vi "Yscaling_raw.vi"(6 "Scaling?":bool, 10 "Y":dbl, 11 "Plane Height (m)":dbl) -> (3 "y scaled (m)":dbl, 4 "Zpos Graph (nm)":cluster{dbl, "function return":dbl})   [LabVIEW 2019]
uses:
  GlobalClicksHeight_raw.vi
  2017 FINAL/Users/brarlab/Documents/GitHub/LabView-VIs/nanonis vers/Program Files/National Instruments/LabVIEW 2019/user.lib/HapticSTM/HapticSTM.lvlib
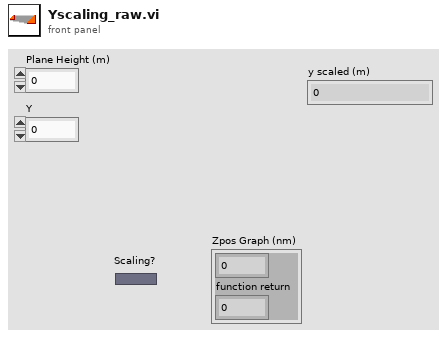
[diagram p1: front panel]
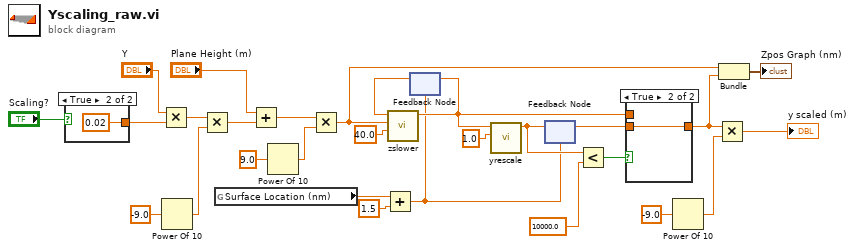
[diagram p0: block diagram]
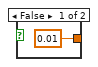
[diagram p2: hidden frame]
diagram:
  n1 = case shown="True" "Scaling?" {
    tunnel: [0.01 ("y") 0.02 ("y")] -> w1
    frame False {
    }
    frame True {
    }
  }
  n2 = Multiply(x="Y", y=w1) -> (x*y=w24:dbl)
  n3 = Power Of 10(x=-9.0) -> (10^x=w23:dbl)
  n4 = Multiply(x=w24, y=w23) -> (x*y=w25:dbl)
  n5 = global read "GlobalClicksHeight_raw.vi" "Surface Location (nm)"() -> (w6:dbl)
  n6 = Add(x="Plane Height (m)", y=w25) -> (x+y=w28:dbl)
  n7 = Power Of 10(x=9.0) -> (10^x=w27:dbl)
  n8 = Multiply(x=w28, y=w27) -> (x*y=w9:dbl)
  n9 = Add(x=w6, y=1.5) -> (x+y=w4:dbl)
  n10 = feedback #1(w4) -> (w11:dbl)
  n11 = call "zslower.vi"("maxvel"=40.0, "labview_zpos_write"=w9, "nanonis_zpos_read"=w11) -> ("function return"=w7:dbl)  [unwired: 8 in]
  n12 = feedback-in #1(w7) -> ()
  n13 = call "yrescale.vi"("scalingfactor"=1.0, "ylabview"=w7) -> ("function return"=w8:dbl)  [unwired: 9 in]
  n14 = feedback-in #2(w8) -> ()
  n15 = feedback #2(w4) -> (w13:dbl)
  n16 = Less?(x=w8, y=10000.0) -> (x < y?=w14:bool)
  n17 = case shown="True" w14 {
    tunnel: [w31 w32] -> w3
    tunnel: w13 -> [_ w32]
    tunnel: w7 -> [w31 _]
    frame False {
    }
    frame True {
    }
  }
  n18 = Power Of 10(x=-9.0) -> (10^x=w18:dbl)
  n19 = Multiply(x=w3, y=w18) -> (x*y=→"y scaled (m)":dbl)
  n20 = Bundle(w9, "function return"=w3) -> (→"Zpos Graph (nm)":cluster{dbl, "function return":dbl})  [unwired: 1 in]
